vi "Input_String_Dialog.vi"(2 "Value":string, 3 "Message to user":string) -> (0 "Ok Out":bool, 1 "Output string":string)   [LabVIEW 2010]
panel:
  in  "Value 2":string
  out "Message to user 2":string
  in  "OK":bool
  in  "Cancel":bool
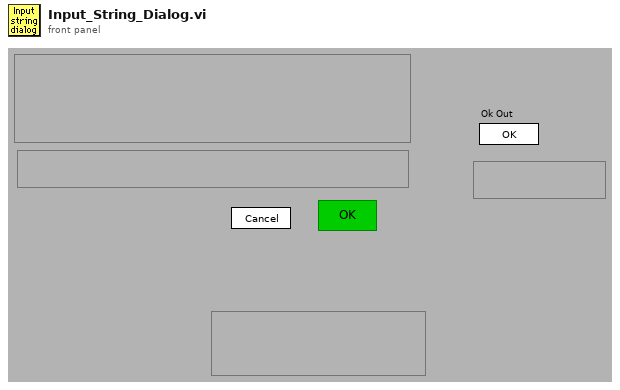
[diagram p1: front panel]
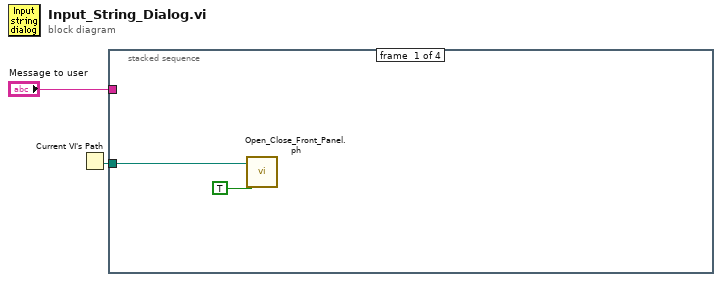
[diagram p0: block diagram]
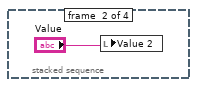
[diagram p2: hidden frame]
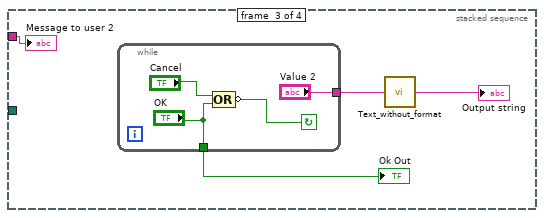
[diagram p3: hidden frame]
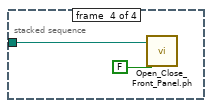
[diagram p4: hidden frame]
diagram:
  n1 = Current VI's Path() -> (path=w2:path)
  n2 = stacked-sequence {
    tunnel: w2 -> [w3 _ _ w14]
    tunnel: "Message to user" -> [_ _ w6 _]
    frame #0 {
      n3 = call "Open_Close_Front_Panel.ph.vi"("Front Panel Window:Open"=TRUE, "VI path"=w3) -> ()  [unwired: 2 out]
    }
    frame #1 {
      n4 = local write "Value 2"("Value") -> ()
    }
    frame #2 {
      n5 = while {
        tunnel: ["OK"] -> w9
        tunnel: ["Value 2"] -> w8
        stop <- w12 continue-if-true
        n6 = Compound Arithmetic op=OR("Cancel", "OK") -> (invert w12:bool)
      }
      "Ok Out" <- w9
      n7 = call "Text_without_format.vi"("Input string"=w8) -> ("Output string"=→"Output string":string)
      "Message to user 2" <- w6
    }
    frame #3 {
      n8 = call "Open_Close_Front_Panel.ph.vi"("Front Panel Window:Open"=FALSE, "VI path"=w14) -> ()  [unwired: 2 out]
    }
  }
